vi "Write applicationElements.vi"(10 "applicationElements":T1, 11 "Model in":refnum<class "Model.lvclass">) -> (3 "Model out":refnum<class "Model.lvclass">)   [LabVIEW 2013, in "Model.lvclass"]
uses:
  Model.lvclass
  ApplicationElements/ApplicationElements.ctl
  ApplicationElements/SystemController/SystemController.lvclass
  ApplicationElements/TestMonitor/TestMonitor.lvclass
  ApplicationElements/StiffnessMonitor/StiffnessMonitor.lvclass
  ApplicationElements/Thermocouple/Thermocouple.lvclass
  ApplicationElements/Log/TestDataLog/TestDataLog.lvclass
  ApplicationElements/Log/StiffnessLog/StiffnessLog.lvclass
  ApplicationElements/DistanceGaugeTC/DistanceGaugeTC.lvclass
  ApplicationElements/EncoderReaderTC/EncoderReaderTC.lvclass
  ApplicationElements/StepperMotorTC/StepperMotorTC.lvclass
  ApplicationElements/ForceSensorCalculatorTC/ForceSensorCalculatorTC.lvclass
  ApplicationElements/EncoderConverterTC/EncoderConverterTC.lvclass
  Model.lvclass/Model.ctl
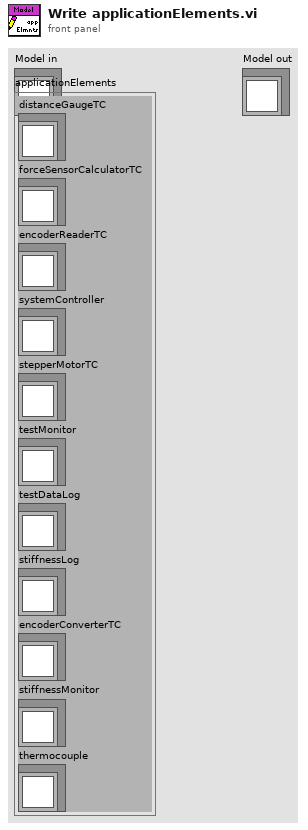
[diagram p1: front panel]
types:
  T1 = typedef "ApplicationElements.ctl" = cluster{"distanceGaugeTC":refnum<class "DistanceGaugeTC.lvclass">, "forceSensorCalculatorTC":refnum<class "ForceSensorCalculatorTC.lvclass">, "encoderReaderTC":refnum<class "EncoderReaderTC.lvclass">, "systemController":refnum<class "SystemController.lvclass">, "stepperMotorTC":refnum<class "StepperMotorTC.lvclass">, "testMonitor":refnum<class "TestMonitor.lvclass">, "testDataLog":refnum<class "TestDataLog.lvclass">, "stiffnessLog":refnum<class "StiffnessLog.lvclass">, "encoderConverterTC":refnum<class "EncoderConverterTC.lvclass">, "stiffnessMonitor":refnum<class "StiffnessMonitor.lvclass">, "thermocouple":refnum<class "Thermocouple.lvclass">}
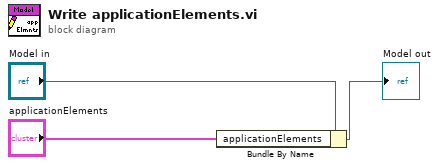
[diagram p0: block diagram]
diagram:
  n1 = Bundle By Name(cluster="Model in", "applicationElements"="applicationElements") -> (→"Model out":refnum<class "Model.lvclass">)
